vi "Read Measurement (Harmonic).vi"(0 "VISA resource name":refnum<visa-resource-name>, 5 "Timeout (10000 ms)":i32=10000 format="%.0g", 7 "Read Option (1)":i32=1 format="%.0g", 9 "Data Type (0:Total Harmonic Distortion)":i32(ring) items=["Total Harmonic Distortion", "Frequency", "Specified Harmonic Amplitude"], 11 "error in (no error)":errorcluster) -> (4 "VISA resource name out":refnum<visa-resource-name>, 6 "Measurement Data":dbl[](array[numeric]), 15 "error out":errorcluster)   [LabVIEW 2018, in "Agilent MXA Series.lvlib"]
doc: "Reads the harmonic measurement result from the spectrum analyzer."
uses:
  Agilent MXA Series.lvlib
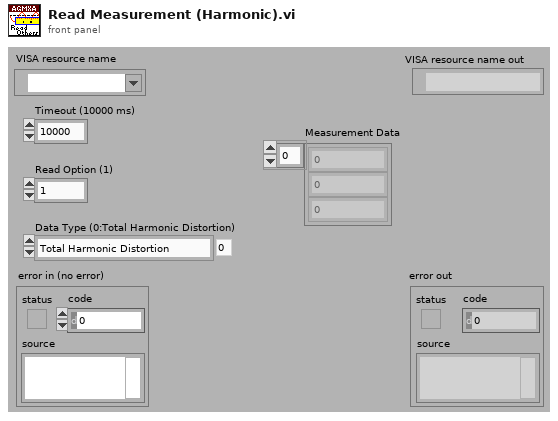
[diagram p1: front panel]
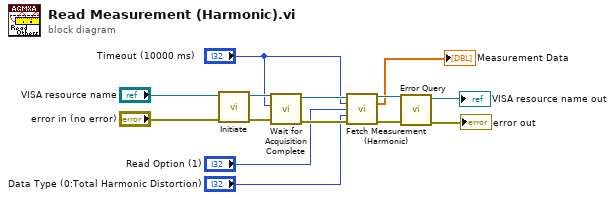
[diagram p0: block diagram]
diagram:
  n1 = call "Initiate.vi"("error in (no error)"="error in (no error)", "VISA resource name"="VISA resource name") -> ("error out"=w11:errorcluster, "VISA resource name out"=w12:refnum<visa-resource-name>)  [unwired: 8 in]
  n2 = call "Wait for Acquisition Complete.vi"("error in (no error)"=w11, "Maximum Time (10000)"="Timeout (10000 ms)", "VISA resource name"=w12) -> ("error out"=w9:errorcluster, "VISA resource name out"=w10:refnum<visa-resource-name>)  [unwired: 7 in]
  n3 = call "Fetch Measurement (Harmonic).vi"("VISA resource name"=w10, "Timeout (10000 ms)"="Timeout (10000 ms)", "Fetch Option (1)"="Read Option (1)", "Data Type (0:Total Harmonic Distortion)"="Data Type (0:Total Harmonic Distortion)", "error in (no error)"=w9) -> ("VISA resource name out"=w7:refnum<visa-resource-name>, "Measurement Data"=→"Measurement Data":dbl[], "error out"=w6:errorcluster)  [unwired: 8 in]
  n4 = call "Error Query.vi"("error in (no error)"=w6, "VISA resource name"=w7) -> ("error out"=→"error out":errorcluster, "VISA resource name out"=→"VISA resource name out":refnum<visa-resource-name>)  [unwired: 6 in, 2 out]
